vi "onDestroy.vi"(8 "error in (no error)":errorcluster, 11 "Server in":refnum<class "Server.lvclass">) -> (0 "error out":errorcluster, 3 "Server out":refnum<class "Server.lvclass">)   [LabVIEW 2013, in "MQTT Server.lvlib" / "Server.lvclass"]
uses:
  Server.lvclass
  <vilib>/LabVIEW Open Source Project/MQTT Connection/MQTT_Base/Base Class/MQTT_Base.lvclass
  Server.lvclass/Server.ctl
  StoredSessions/StoredSessions.lvclass
  Subscription/Subscription.lvclass
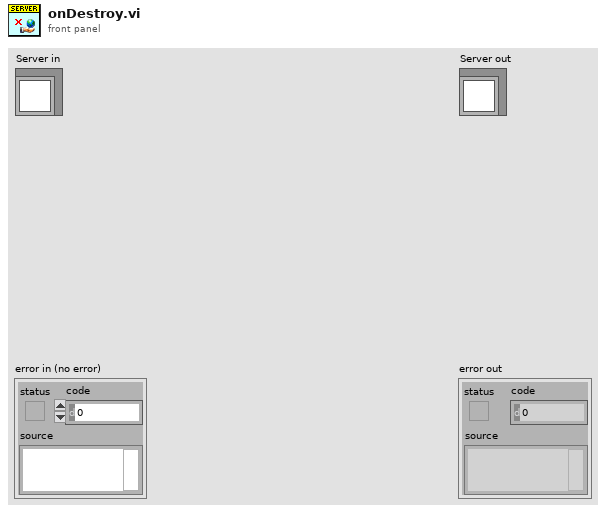
[diagram p1: front panel]
types:
  T1 = typedef "MQTT Server.lvlib/Server.lvclass/SessionRef -- cluster.ctl" = cluster{"ClientID":string, "SessionMailbox":refnum<queue>}
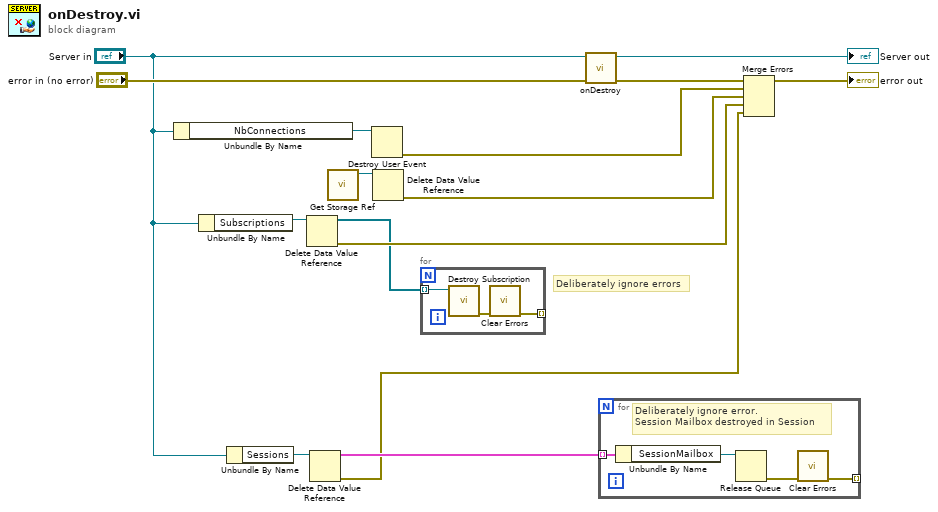
[diagram p0: block diagram]
diagram:
  # "Deliberately ignore errors"
  n1 = Unbundle By Name("Server in") -> ("NbConnections"=w12:refnum<user-event>)
  n2 = Unbundle By Name("Server in") -> ("Subscriptions"=w4:refnum<data-value>)
  n3 = Unbundle By Name("Server in") -> ("Sessions"=w6:refnum<data-value>)
  n4 = Delete Data Value Reference(data value reference=w4) -> (data value=w1:refnum<class "Subscription.lvclass">[], error out=w3:errorcluster)  [unwired: 1 in]
  n5 = Delete Data Value Reference(data value reference=w6) -> (data value=w7:T1[], error out=w2:errorcluster)  [unwired: 1 in]
  n6 = call "Get Storage Ref.vi"() -> ("Storage"=w14:refnum<data-value>)  [unwired: 11 in]
  n7 = Destroy User Event(user event=w12) -> (error out=w8:errorcluster)  [unwired: 1 in]
  n8 = Delete Data Value Reference(data value reference=w14) -> (error out=w13:errorcluster)  [unwired: 1 in, 1 out]
  n9 = for {
    tunnel: w1 -> [w18] mode=indexing
    tunnel: [w16] -> _ mode=indexing
    n10 = call "Destroy Subscription.vi"("Subscription in"=w18) -> ("error out"=w17:errorcluster)  [unwired: 9 in, 1 out]
    n11 = call <vilib>:"Clear Errors.vi"("error in (no error)"=w17) -> ("error out"=w16:errorcluster)  [unwired: 6 in]
  }
  n12 = call-parent "onDestroy.vi"("error in (no error)"="error in (no error)", "MQTT_Base in"="Server in") -> ("error out"=w10:errorcluster, "MQTT_Base out"=→"Server out":refnum<class "Server.lvclass">)  [unwired: 8 in]
  n13 = for {
    tunnel: w7 -> [w22] mode=indexing
    tunnel: [w19] -> _ mode=indexing
    # "Deliberately ignore error.\nSession Mailbox destroyed in Session"
    n14 = Unbundle By Name(w22) -> ("SessionMailbox"=w21:refnum<queue>)
    n15 = Release Queue(queue=w21) -> (error out=w20:errorcluster)  [unwired: 2 in, 2 out]
    n16 = call <vilib>:"Clear Errors.vi"("error in (no error)"=w20) -> ("error out"=w19:errorcluster)  [unwired: 6 in]
  }
  n17 = Merge Errors(w10, w8, w13, w3, w2) -> (→"error out":errorcluster)
